vi "Write D Full System Cal.vi"(6 "Cal File Path":path, 8 "error in (no error)":errorcluster, 9 "Model":string, 10 "Cal Serial Number":string, 11 "Cal DateDBL":dbl) -> (0 "error out":errorcluster)   [LabVIEW 2011]
uses:
  Module Cal File Section.ctl
  <vilib>/Utility/config.llb/Write Key (String).vi
  <vilib>/Utility/config.llb/Write Key (Double).vi
  WebEngine/LIB/HW Global D.vi
  <vilib>/Utility/config.llb/NI_LVConfig.lvlib
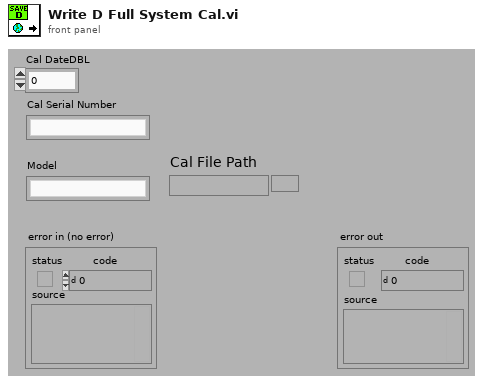
[diagram p1: front panel]
types:
  T1 = typedef "Module Cal File Section.ctl" = enum16{"CARRIER1 VS FREQ", "CARRIER2 VS FREQ", "PAD1 VS FREQUENCY", "PAD2 VS FREQUENCY", "RX POWER VS FREQUENCY", "PORT 3 VS ATTENUATION", "PORT 3 VS FREQUENCY", "HIGH POWER PAD VS FREQUENCY", "D1 VS ATTENUATION", "D1 VS FREQUENCY", "D2 VS ATTENUATION", "D2 VS FREQUENCY", "D1 LOSS VS FREQUENCY", "D2 LOSS VS FREQUENCY", "RX REVERSE", "RX FORWARD", "RX AUXILIARY", "TXA", "TXB", "TXC", "RXA", "RXB", "RXC", "RXD", "RXE", "RXF"}
  T2 = typedef "NI_LVConfig.lvlib/Config Data RefNum.ctl" = refnum<k1>
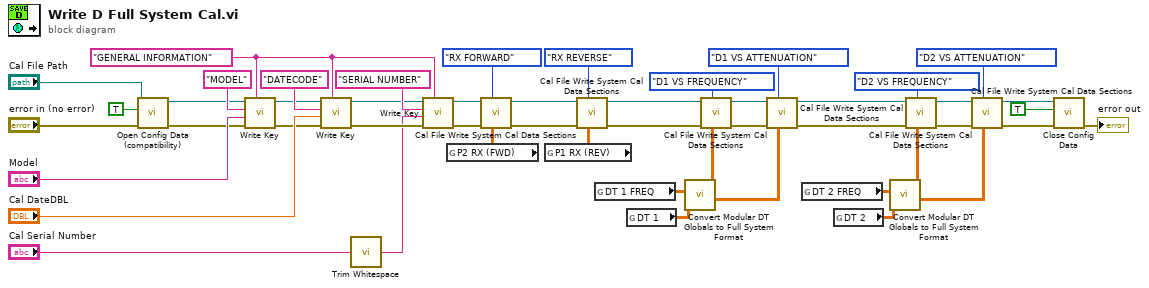
[diagram p0: block diagram]
diagram:
  w26 = "GENERAL INFORMATION"
  n1 = call <vilib>:"Open Config Data (compatibility).vi"("error in (no error)"="error in (no error)", "create file if necessary (T)"=TRUE, "configuration file path"="Cal File Path") -> ("error out"=w20:errorcluster, "refnum"=w24:T2)  [unwired: 6 in, 1 out]
  n2 = call-poly <vilib>:"Write Key.vi"("section"=w26, "error in (no error)"=w20, "value"="Model", "key"="MODEL", "refnum"=w24) -> ("error out"=w22:errorcluster, "refnum out"=w23:T2)  [unwired: 4 in, 1 out]
  n3 = call-poly <vilib>:"Write Key.vi"("section"=w26, "error in (no error)"=w22, "value"="Cal DateDBL", "key"="DATECODE", "refnum"=w23) -> ("error out"=w32:errorcluster, "refnum out"=w31:T2)  [unwired: 4 in, 1 out]
  n4 = call <vilib>:"Trim Whitespace.vi"("string"="Cal Serial Number") -> ("trimmed string"=w19:string)  [unwired: 1 in]
  n5 = call-poly <vilib>:"Write Key.vi"("section"=w26, "error in (no error)"=w32, "value"=w19, "key"="SERIAL NUMBER", "refnum"=w31) -> ("error out"=w36:errorcluster, "refnum out"=w37:T2)  [unwired: 4 in, 1 out]
  n6 = global read "HW Global D.vi" "P2 RX (FWD)"() -> (w28:dbl[][])
  n7 = call "Cal File Write System Cal Data Sections.vi"("DATA"=w28, "DATA SECTION"=Module_Cal_File_Section."RX FORWARD", "error in (no error)"=w36, "Cal Ref"=w37) -> ("error out"=w38:errorcluster, "Cal Ref out"=w39:T2)  [unwired: 6 in]
  n8 = global read "HW Global D.vi" "P1 RX (REV)"() -> (w41:dbl[][])
  n9 = call "Cal File Write System Cal Data Sections.vi"("DATA"=w41, "DATA SECTION"=Module_Cal_File_Section."RX REVERSE", "error in (no error)"=w38, "Cal Ref"=w39) -> ("error out"=w18:errorcluster, "Cal Ref out"=w17:T2)  [unwired: 6 in]
  n10 = global read "HW Global D.vi" "DT 1 FREQ"() -> (w7:dbl[][])
  n11 = global read "HW Global D.vi" "DT 1"() -> (w8:dbl[][])
  n12 = call "Convert Modular DT Globals to Full System Format.vi"("DT in"=w8, "DT FREQ in"=w7) -> ("DT out"=w5:dbl[][], "DT FREQ out"=w6:dbl[][])  [unwired: 8 in]
  n13 = call "Cal File Write System Cal Data Sections.vi"("DATA"=w6, "DATA SECTION"=Module_Cal_File_Section."D1 VS FREQUENCY", "error in (no error)"=w18, "Cal Ref"=w17) -> ("error out"=w15:errorcluster, "Cal Ref out"=w16:T2)  [unwired: 6 in]
  n14 = call "Cal File Write System Cal Data Sections.vi"("DATA"=w5, "DATA SECTION"=Module_Cal_File_Section."D1 VS ATTENUATION", "error in (no error)"=w15, "Cal Ref"=w16) -> ("error out"=w14:errorcluster, "Cal Ref out"=w13:T2)  [unwired: 6 in]
  n15 = global read "HW Global D.vi" "DT 2 FREQ"() -> (w4:dbl[][])
  n16 = global read "HW Global D.vi" "DT 2"() -> (w3:dbl[][])
  n17 = call "Convert Modular DT Globals to Full System Format.vi"("DT in"=w3, "DT FREQ in"=w4) -> ("DT out"=w1:dbl[][], "DT FREQ out"=w2:dbl[][])  [unwired: 8 in]
  n18 = call "Cal File Write System Cal Data Sections.vi"("DATA"=w2, "DATA SECTION"=Module_Cal_File_Section."D2 VS FREQUENCY", "error in (no error)"=w14, "Cal Ref"=w13) -> ("error out"=w12:errorcluster, "Cal Ref out"=w11:T2)  [unwired: 6 in]
  n19 = call "Cal File Write System Cal Data Sections.vi"("DATA"=w1, "DATA SECTION"=Module_Cal_File_Section."D2 VS ATTENUATION", "error in (no error)"=w12, "Cal Ref"=w11) -> ("error out"=w9:errorcluster, "Cal Ref out"=w10:T2)  [unwired: 6 in]
  n20 = call <vilib>:"Close Config Data.vi"("error in (no error)"=w9, "write file if changed (T)"=TRUE, "refnum"=w10) -> ("error out"=→"error out":errorcluster)  [unwired: 8 out]
